vi "DSO1072B_FeatchWaveCW.vi"(11 "VISA resource name In":refnum<visa-resource-name>="USB0::0x0957::0x0588::CN55040452::INSTR") -> (0 "Avg4V8":dbl, 1 "Avg2V9":dbl, 2 "Avg2V1":dbl, 3 "Avg1V3":dbl, 5 "XY Graph CH1":cluster{"Numeric":dbl, "Numeric":dbl}[](graph))   [LabVIEW 2018]
panel:
  out "OutCompare 2":bool
  out "OutCompare 3":bool
  out "OutCompare 4":bool
  out "OutCompare":bool
  out "sum":dbl
  out "subarray":dbl[](array[numeric])
  out "x+y":i32
  out "StartIndeXof2V1":i32
  out "StartIndeXof1V3":i32
  out "StartIndeXof2V9":i32
  out "StartIndeXof4V8":i32
  out "Y-DataCH1":dbl[](array[numeric])
  out "X-DataCH1":dbl[](array[numeric])
  out "yreference":dbl
  out "yorigin":dbl
  out "yincrement":dbl
  out "xreference":dbl
  out "xorigin":dbl
  out "xincrement":dbl format="%#_6f"
  out "NumberOfPoint":i32
  out "<yref>":string
  out "<yorigi>":string
  out "<yinc>":string
  out "<xref>":string
  out "<xorigi>":string
  out "<xinc>":string
  out "<count>":string
  out "<points>":string
  out "<type>":string
  out "<format>":string
  out ":WAV:PRE":string
  out "length":i32
  out "ByteFormatDataCH1":string
  out "data_valueCH1":u8[](array[numeric])
  out "ByteArrayCH1":u8[](array[numeric]) format="%x"
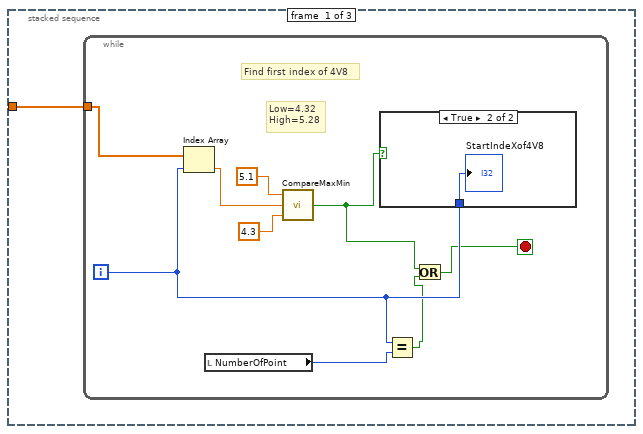
[diagram p3: hidden frame]
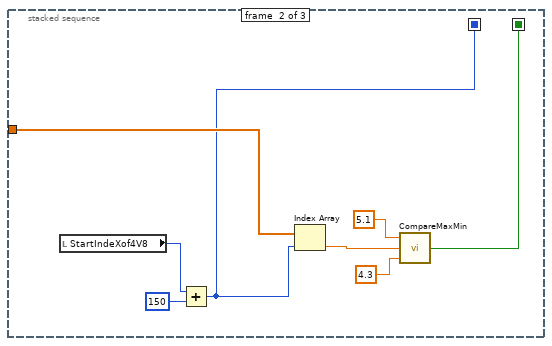
[diagram p5: hidden frame]
diagram:
  n1 = flat-sequence {
    tunnel: ["VISA resource name In"] -> w9
    tunnel: [w23] -> w10
    tunnel: w9 -> [w23]
    tunnel: [w28] -> w11
    tunnel: w10 -> [w28]
    tunnel: w11 -> [w66]
    tunnel: [w90] -> w8
    tunnel: w8 -> [w134]
    tunnel: [w134] -> w7
    tunnel: w7 -> [w137]
    tunnel: [w137] -> w6
    tunnel: w6 -> [w154]
    tunnel: [w154] -> w5
    tunnel: w5 -> [w161]
    tunnel: [w161] -> w4
    tunnel: w4 -> [w178]
    tunnel: [w178] -> w3
    tunnel: w3 -> [w185]
    tunnel: [w185] -> w2
    tunnel: w2 -> [w202]
    tunnel: [w202] -> w1
    tunnel: [w214] -> _
    tunnel: w1 -> [w214]
    frame #0 {
      n2 = Initialize Array(0.0 ("element"), 20480 ("dimension size")) -> (→"Y-DataCH1" →"X-DataCH1":dbl[])
    }
    frame #1 {
      n3 = Wait (ms)(milliseconds to wait=u32 10) -> ()  [unwired: 1 out]
    }
    frame #2 {
      n4 = call "DSO1072B_WaveformCMD1.vi"("AutoRead?"=TRUE, "Delay(mS)"=u32 500, "byte count"=u32 20480, "ManualCMD?"=FALSE, "DSO1072B CMD"=":WAV:DATA? CHAN2", "VISA resource name In"="VISA resource name In") -> ("read buffer"=→"ByteFormatDataCH1":string)  [unwired: 3 in, 2 out]
    }
    frame #3 {
      n5 = case shown="True" TRUE {
        frame False {
        }
        frame True {
          n6 = local read "ByteFormatDataCH1"() -> (w26:string)
          n7 = String To Byte Array(string=w26) -> (unsigned byte array=→"ByteArrayCH1":u8[])
          n8 = String Length(string=w26) -> (length=→"length":i32)
        }
      }
    }
    frame #4 {
      (unwired) 10 ("index")
      w31 = 10 ("index")
      n9 = local read "length"() -> (w32:i32)
      n10 = local read "ByteArrayCH1"() -> (w33:u8[])
      n11 = Subtract(x=w32, y=w31) -> (x-y=w30:i32)
      "NumberOfPoint" <- w30
      n12 = Array Subset(array=w33, index=w31, length=w30) -> (→"data_valueCH1":u8[])
    }
    frame #5 {
      w47 = "," ("regular expression")
      n13 = call "DSO1072B_WaveformCMD1.vi"("AutoRead?"=TRUE, "Delay(mS)"=u32 100, "byte count"=u32 250, "ManualCMD?"=FALSE, "DSO1072B CMD"=":WAV:PRE?", "VISA resource name In"=w66) -> ("read buffer"=w61:string)  [unwired: 3 in, 2 out]
      ":WAV:PRE" <- w61
      n14 = Match Pattern(string=w61, regular expression=w47) -> (before substring=→"<format>":string, after substring=w59:string)  [unwired: 1 in, 2 out]
      n15 = Match Pattern(string=w59, regular expression=w47) -> (before substring=→"<type>":string, after substring=w57:string)  [unwired: 1 in, 2 out]
      n16 = Match Pattern(string=w57, regular expression=w47) -> (before substring=→"<points>":string, after substring=w55:string)  [unwired: 1 in, 2 out]
      n17 = Match Pattern(string=w55, regular expression=w47) -> (before substring=→"<count>":string, after substring=w53:string)  [unwired: 1 in, 2 out]
      n18 = Match Pattern(string=w53, regular expression=w47) -> (before substring=w46:string, after substring=w52:string)  [unwired: 1 in, 2 out]
      "<xinc>" <- w46
      n19 = Match Pattern(string=w52, regular expression=w47) -> (before substring=w44:string, after substring=w51:string)  [unwired: 1 in, 2 out]
      "<xorigi>" <- w44
      n20 = Fract/Exp String To Number(string=w46) -> (number=→"xincrement":dbl)  [unwired: 3 in, 1 out]
      n21 = Match Pattern(string=w51, regular expression=w47) -> (before substring=w41:string, after substring=w50:string)  [unwired: 1 in, 2 out]
      "<xref>" <- w41
      n22 = Fract/Exp String To Number(string=w44) -> (number=→"xorigin":dbl)  [unwired: 3 in, 1 out]
      n23 = Match Pattern(string=w50, regular expression=w47) -> (before substring=w39:string, after substring=w49:string)  [unwired: 1 in, 2 out]
      "<yinc>" <- w39
      n24 = Fract/Exp String To Number(string=w41) -> (number=→"xreference":dbl)  [unwired: 3 in, 1 out]
      n25 = Fract/Exp String To Number(string=w39) -> (number=→"yincrement":dbl)  [unwired: 3 in, 1 out]
      n26 = Match Pattern(string=w49, regular expression=w47) -> (before substring=w37:string, after substring=w48:string)  [unwired: 1 in, 2 out]
      "<yorigi>" <- w37
      n27 = Match Pattern(string=w48, regular expression=w47) -> (before substring=w36:string)  [unwired: 1 in, 3 out]
      "<yref>" <- w36
      n28 = Fract/Exp String To Number(string=w37) -> (number=→"yorigin":dbl)  [unwired: 3 in, 1 out]
      n29 = Fract/Exp String To Number(string=w36) -> (number=→"yreference":dbl)  [unwired: 3 in, 1 out]
    }
    frame #6 {
      # "(YREFerence - data_value)*YINCrement - YORigin"
      # "XORigin + (data_index * XINCrement)"
      n30 = local read "data_valueCH1"() -> (w67:u8[])
      n31 = while {
        tunnel: w67 -> [w89]
        i -> [w71]
        stop <- w73 stop-if-true
        # "(YREFerence – data_value) * YINCrement -YORigin"
        # "XORigin + (data_index * XINCrement)"
        n32 = local read "NumberOfPoint"() -> (w70:i32)
        n33 = local read "yreference"() -> (w82:dbl)
        n34 = local read "yincrement"() -> (w79:dbl)
        n35 = Subtract(x=w70, y=2000) -> (x-y=w68:i32)
        n36 = Index Array(array=w89, index=w71) -> (element=w81:u8)
        n37 = local read "yorigin"() -> (w77:dbl)
        n38 = Equal?(x=w71, y=w68) -> (x = y?=w73:bool)
        n39 = Subtract(x=w82, y=w81) -> (x-y=w80:dbl)
        n40 = local read "xincrement"() -> (w86:dbl)
        n41 = Multiply(x=w80, y=w79) -> (x*y=w78:dbl)
        n42 = Subtract(x=w78, y=w77) -> (x-y=w76:dbl)
        n43 = local read "xorigin"() -> (w88:dbl)
        n44 = Multiply(x=w71, y=w86) -> (x*y=w87:dbl)
        n45 = local read "X-DataCH1"() -> (w85:dbl[])
        n46 = Add(x=w88, y=w87) -> (x+y=w84:dbl)
        n47 = local read "Y-DataCH1"() -> (w83:dbl[])
        n48 = Insert Into Array(array=w85, index=w71, new element=w84) -> (w75:dbl[])
        n49 = Insert Into Array(array=w83, index=w71, new element=w76) -> (w74:dbl[])
        n50 = Build Cluster Array(w75, w74) -> (→"XY Graph CH1":cluster{"Numeric":dbl, "Numeric":dbl}[])
        n51 = local write "X-DataCH1"(w75) -> ()
        n52 = local write "Y-DataCH1"(w74) -> ()
      }
    }
    frame #7 {
      n53 = local read "Y-DataCH1"() -> (w90:dbl[])
      n54 = stacked-sequence {
        seq-local: [_ w104 _] -> [_ _ w112]
        seq-local: [_ w102 _] -> [_ _ w110]
        tunnel: w90 -> [w91 w108 w111]
        frame #0 {
          n55 = while {
            tunnel: w91 -> [w100]
            i -> [w95]
            stop <- w94 stop-if-true
            # "Low=4.32\nHigh=5.28"
            # "Find first index of 4V8"
            n56 = Index Array(array=w100, index=w95) -> (element=w99:dbl)
            n57 = local read "NumberOfPoint"() -> (w96:i32)
            n58 = call "CompareMaxMin.vi"("Min"=4.3, "X"=w99, "Max"=5.1) -> ("OutCompare"=w93:bool)
            n59 = case shown="True" w93 {
              tunnel: w95 -> [_ w101]
              frame False {
              }
              frame True {
                "StartIndeXof4V8" <- w101
              }
            }
            n60 = Equal?(x=w95, y=w96) -> (x = y?=w92:bool)
            n61 = Or(x=w93, y=w92) -> (x .or. y?=w94:bool)
          }
        }
        frame #1 {
          n62 = local read "StartIndeXof4V8"() -> (w103:i32)
          n63 = Add(x=w103, y=150) -> (x+y=w102:i32)
          n64 = Index Array(array=w108, index=w102) -> (element=w105:dbl)
          n65 = call "CompareMaxMin.vi"("Min"=4.3, "X"=w105, "Max"=5.1) -> ("OutCompare"=w104:bool)
        }
        frame #2 {
          n66 = case shown="False" w112 {
            tunnel: w111 -> [w114 _]
            tunnel: w110 -> [w113 _]
            frame False {
              n67 = while {
                tunnel: w114 -> [w125]
                tunnel: w113 -> [w116]
                i -> [w117]
                stop <- w120 stop-if-true
                # "Low=4.32\nHigh=5.28"
                # "Find first index of 4V8"
                n68 = Add(x=w117, y=w116) -> (x+y=w115:i32)
                n69 = Index Array(array=w125, index=w115) -> (element=w124:dbl)
                n70 = local read "NumberOfPoint"() -> (w121:i32)
                n71 = call "CompareMaxMin.vi"("Min"=4.3, "X"=w124, "Max"=5.1) -> ("OutCompare"=w119:bool)
                n72 = case shown="True" w119 {
                  tunnel: w115 -> [_ w126]
                  frame False {
                  }
                  frame True {
                    n73 = local write "StartIndeXof4V8"(w126) -> ()
                  }
                }
                n74 = Equal?(x=w115, y=w121) -> (x = y?=w118:bool)
                n75 = Or(x=w119, y=w118) -> (x .or. y?=w120:bool)
              }
            }
            frame True {
            }
          }
        }
      }
    }
    frame #8 {
      (unwired) 100 ("y")
      w131 = 50 ("y")
      # "997"
      # "975"
      # "100 point to attain stable 4V8 value"
      n76 = local read "StartIndeXof4V8"() -> (w132:i32)
      n77 = Add(x=w132, y=w131) -> (x+y=→"x+y":i32)
      n78 = Array Subset(array=w134, index=w132, length=w131) -> (w136:dbl[])
      "subarray" <- w136
      n79 = Add Array Elements(numeric array=w136) -> (sum=w135:dbl)
      "sum" <- w135
      n80 = Divide(x=w135, y=w131) -> (x/y=w127:dbl)
      "Avg4V8" <- w127
      n81 = call "CompareMaxMin.vi"("Min"=4.32, "X"=w127, "Max"=5.28) -> ("OutCompare"=→"OutCompare":bool)
    }
    frame #9 {
      n82 = while {
        tunnel: w137 -> [w148]
        i -> [w144]
        stop <- w140 stop-if-true
        # "Low=2.61\nHigh=3.19"
        # "Find first index of 2V9"
        n83 = local read "StartIndeXof4V8"() -> (w143:i32)
        n84 = Add(x=w144, y=w143) -> (x+y=w138:i32)
        n85 = Index Array(array=w148, index=w138) -> (element=w147:dbl)
        n86 = local read "NumberOfPoint"() -> (w141:i32)
        n87 = call "CompareMaxMin.vi"("Min"=2.6, "X"=w147, "Max"=3.0) -> ("OutCompare"=w139:bool)
        n88 = Equal?(x=w138, y=w141) -> (x = y?=w142:bool)
        n89 = case shown="True" w139 {
          tunnel: w138 -> [_ w149]
          frame False {
          }
          frame True {
            "StartIndeXof2V9" <- w149
          }
        }
        n90 = Or(x=w139, y=w142) -> (x .or. y?=w140:bool)
      }
    }
    frame #10 {
      w156 = 150 ("length")
      # "100 point to attain stable 4V8 value"
      n91 = local read "StartIndeXof2V9"() -> (w155:i32)
      n92 = Add(x=w155, y=100) -> (x+y=w159:i32)
      n93 = Array Subset(array=w154, index=w159, length=w156) -> (w158:dbl[])
      n94 = Add Array Elements(numeric array=w158) -> (sum=w157:dbl)
      n95 = Divide(x=w157, y=w156) -> (x/y=w150:dbl)
      "Avg2V9" <- w150
      n96 = call "CompareMaxMin.vi"("Min"=2.61, "X"=w150, "Max"=3.19) -> ("OutCompare"=→"OutCompare 4":bool)
    }
    frame #11 {
      n97 = while {
        tunnel: w161 -> [w172]
        i -> [w168]
        stop <- w164 stop-if-true
        # "Low=1.17\nHigh=1.43"
        # "Find first index of 1V3"
        n98 = local read "StartIndeXof2V9"() -> (w167:i32)
        n99 = Add(x=w168, y=w167) -> (x+y=w162:i32)
        n100 = Index Array(array=w172, index=w162) -> (element=w171:dbl)
        n101 = local read "NumberOfPoint"() -> (w165:i32)
        n102 = call "CompareMaxMin.vi"("Min"=1.2, "X"=w171, "Max"=1.55) -> ("OutCompare"=w163:bool)
        n103 = case shown="True" w163 {
          tunnel: w162 -> [_ w173]
          frame False {
          }
          frame True {
            "StartIndeXof1V3" <- w173
          }
        }
        n104 = Equal?(x=w162, y=w165) -> (x = y?=w166:bool)
        n105 = Or(x=w163, y=w166) -> (x .or. y?=w164:bool)
      }
    }
    frame #12 {
      w183 = 150 ("length")
      # "100 point to attain stable 4V8 value"
      n106 = local read "StartIndeXof1V3"() -> (w184:i32)
      n107 = Add(x=w184, y=100) -> (x+y=w180:i32)
      n108 = Array Subset(array=w178, index=w180, length=w183) -> (w181:dbl[])
      n109 = Add Array Elements(numeric array=w181) -> (sum=w182:dbl)
      n110 = Divide(x=w182, y=w183) -> (x/y=w174:dbl)
      "Avg1V3" <- w174
      n111 = call "CompareMaxMin.vi"("Min"=1.17, "X"=w174, "Max"=1.43) -> ("OutCompare"=→"OutCompare 3":bool)
    }
    frame #13 {
      n112 = while {
        tunnel: w185 -> [w196]
        i -> [w192]
        stop <- w188 stop-if-true
        # "Low=1.89\nHigh=2.31"
        # "Find first index of 1V3"
        n113 = local read "StartIndeXof1V3"() -> (w191:i32)
        n114 = Add(x=w192, y=w191) -> (x+y=w186:i32)
        n115 = Index Array(array=w196, index=w186) -> (element=w195:dbl)
        n116 = local read "NumberOfPoint"() -> (w190:i32)
        n117 = call "CompareMaxMin.vi"("Min"=1.9, "X"=w195, "Max"=2.3) -> ("OutCompare"=w187:bool)
        n118 = case shown="True" w187 {
          tunnel: w186 -> [_ w197]
          frame False {
          }
          frame True {
            "StartIndeXof2V1" <- w197
          }
        }
        n119 = Equal?(x=w186, y=w190) -> (x = y?=w189:bool)
        n120 = Or(x=w187, y=w189) -> (x .or. y?=w188:bool)
      }
    }
    frame #14 {
      w204 = 150 ("length")
      # "100 point to attain stable 4V8 value"
      n121 = local read "StartIndeXof2V1"() -> (w203:i32)
      n122 = Add(x=w203, y=100) -> (x+y=w207:i32)
      n123 = Array Subset(array=w202, index=w207, length=w204) -> (w206:dbl[])
      n124 = Add Array Elements(numeric array=w206) -> (sum=w205:dbl)
      n125 = Divide(x=w205, y=w204) -> (x/y=w198:dbl)
      "Avg2V1" <- w198
      n126 = call "CompareMaxMin.vi"("Min"=1.89, "X"=w198, "Max"=2.31) -> ("OutCompare"=→"OutCompare 2":bool)
    }
    frame #15 {
      n127 = local read "OutCompare 4"() -> (w212:bool)
      n128 = local read "OutCompare"() -> (w213:bool)
      n129 = local read "OutCompare 3"() -> (w211:bool)
      n130 = local read "OutCompare 2"() -> (w210:bool)
      n131 = Compound Arithmetic op=AND(w213, w212, w211, w210) -> (w209:bool)
      n132 = case shown="False" w209 {
        frame False {
          n133 = Wait (ms)(milliseconds to wait=u32 0) -> ()  [unwired: 1 out]
        }
        frame True {
        }
      }
    }
  }
